vi "AddSig2SelList.vi"(4 "NumSelected":refnum<vi>, 6 "DBCAllSigArry":refnum<vi>, 7 "YaxleNum":i32, 9 "SelectedSigList":refnum<vi>, 10 "Tag":string, 11 "TreeControl输入":refnum<vi>) -> ()   [LabVIEW 2015]
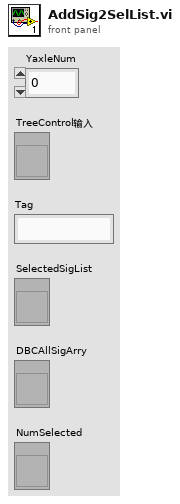
[diagram p1: front panel]
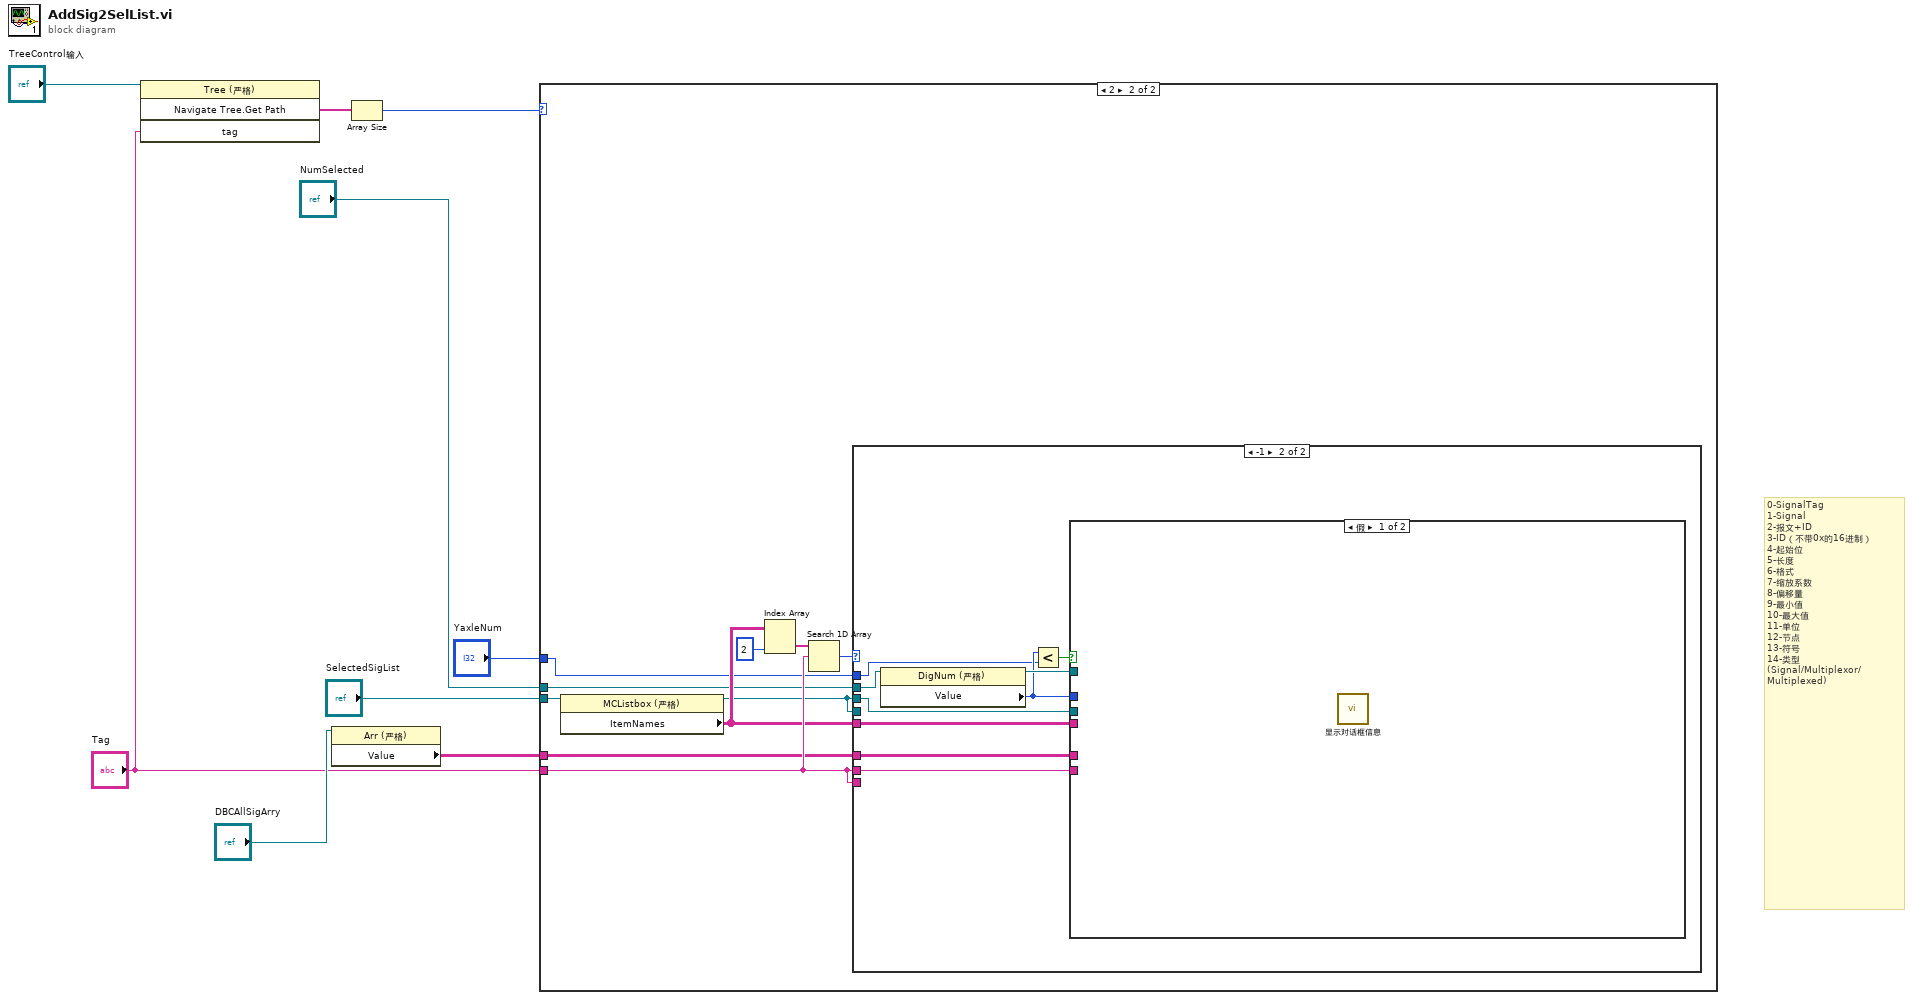
[diagram p0: block diagram]
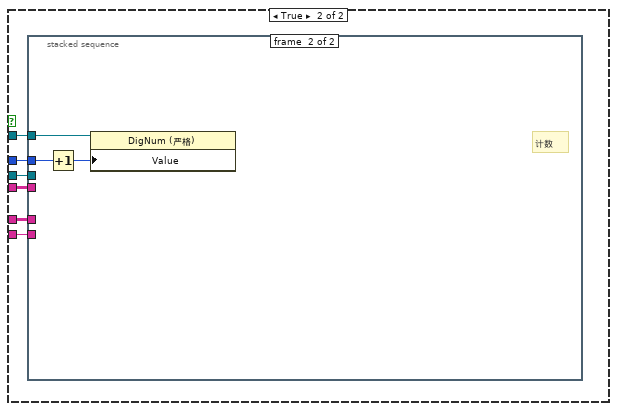
[diagram p4: hidden frame]
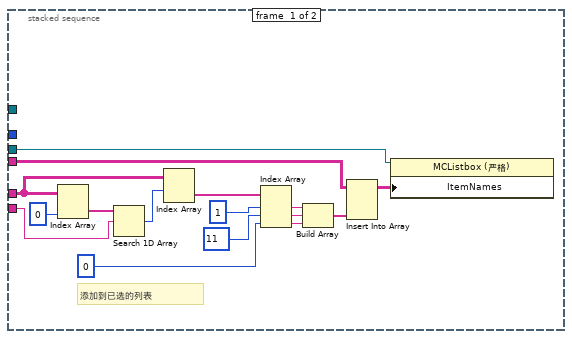
[diagram p5: hidden frame]
diagram:
  # "0-SignalTag\n1-Signal\n2-报文+ID\n3-ID（不带0x的16进制）\n4-起始位\n5-长度\n6-格式\n7-缩放系数\n8-偏移量\n9-最小值\n10-最大值\n11-单位\n12-节点\n13-符号\n14-类型\n(Signal/Multiplexor/\nMultiplexed)"
  n1 = invoke class="Tree (严格)" method="Navigate Tree.Get Path"(reference="TreeControl输入", "tag"="Tag") -> ("Navigate Tree:Get Path"=w3:string[])  [unwired: 2 in, 3 out]
  n2 = property class="Arr (严格)"(reference="DBCAllSigArry") -> ("Value"=w8:string[][])  [unwired: 1 in, 2 out]
  n3 = Array Size(array=w3) -> (size(s)=w4:i32)
  n4 = case shown="2" w4 {
    tunnel: "SelectedSigList" -> [_ w19]
    tunnel: w8 -> [_ w14]
    tunnel: "Tag" -> [_ w15]
    tunnel: "YaxleNum" -> [_ w11]
    tunnel: "NumSelected" -> [_ w10]
    frame 1, Default {
    }
    frame 2 {
      n5 = property on="属性节点" class="MCListbox (严格)"(reference=w19) -> (reference out=w12:refnum<vi>, "ItemNames"=w13:string[][])  [unwired: 1 in, 1 out]
      n6 = Index Array(array=w13, index (col)=2 ("禁用的索引 (列)")) -> (element=w17:string[])  [unwired: 1 in]
      n7 = Search 1D Array(1D array=w17, element=w15) -> (index of element=w16:i32)  [unwired: 1 in]
      n8 = case shown="-1" w16 {
        tunnel: w12 -> [_ _]
        tunnel: w15 -> [_ _]
        tunnel: w14 -> [_ w28]
        tunnel: w15 -> [_ w27]
        tunnel: w13 -> [_ w26]
        tunnel: w12 -> [_ w25]
        tunnel: w11 -> [_ w21]
        tunnel: w10 -> [_ w20]
        frame 0, Default {
        }
        frame -1 {
          n9 = property class="DigNum (严格)"(reference=w20) -> (reference out=w24:refnum<vi>, "Value"=w22:i32)  [unwired: 1 in, 1 out]
          n10 = Less?(x=w22, y=w21) -> (x < y?=w23:bool)
          n11 = case shown="假" w23 {
            tunnel: w28 -> [_ w34]
            tunnel: w27 -> [_ w33]
            tunnel: w26 -> [_ w32]
            tunnel: w25 -> [_ w31]
            tunnel: w24 -> [_ w30]
            tunnel: w22 -> [_ w29]
            frame False {
              n12 = call "显示对话框信息"() -> ()  [unwired: 10 in, 2 out]
            }
            frame True {
              n13 = stacked-sequence {
                tunnel: w34 -> [w35 _]
                tunnel: w33 -> [w39 _]
                tunnel: w32 -> [w37 _]
                tunnel: w31 -> [w36 _]
                tunnel: w30 -> [_ w52]
                tunnel: w29 -> [_ w51]
                frame #0 {
                  # "添加到已选的列表"
                  n14 = Index Array(array=w35, index (col)=0 ("禁用的索引 (列)")) -> (element=w44:string[])  [unwired: 1 in]
                  n15 = Search 1D Array(1D array=w44, element=w39) -> (index of element=w45:i32)  [unwired: 1 in]
                  n16 = Index Array(array=w35, index (row)=w45) -> (element=w46:string[])  [unwired: 1 in]
                  n17 = Index Array(array=w46, index #1=1 ("禁用的索引 (列)"), index #2=11 ("索引 (列)"), index #3=0 ("索引 (列)")) -> (element #1=w47:string, element #2=w48:string, element #3=w49:string)
                  n18 = Build Array(w47, w48, w49) -> (w50:string[])
                  n19 = Insert Into Array(array=w37, new element=w50) -> (w43:string[][])  [unwired: 2 in]
                  n20 = property on="属性节点" class="MCListbox (严格)"(reference=w36, "ItemNames"=w43) -> ()  [unwired: 1 in, 2 out]
                }
                frame #1 {
                  # "计数"
                  n21 = Increment(x=w51) -> (x+1=w53:i32)
                  n22 = property class="DigNum (严格)"(reference=w52, "Value"=w53) -> ()  [unwired: 1 in, 2 out]
                }
              }
            }
          }
        }
      }
    }
  }
